vi "PicoScope6000SetupStreaming.vi"(0 "error in":errorcluster, 1 "Device Info":T2, 2 "handle in":i16, 3 "Acquisition Settings":T3={"Auto Stop"=FALSE, "Desired Sample Interval"=4, "Pre-trigger Samples"=0, "Post-trigger Samples"=1000, "Down-Sample Ratio"=1, "Down-Sample Mode"=0, "Time Units"=2} {"Time Units" items=["Nanoseconds (ns)"=2, "Microseconds (us)"=3, "Milliseconds (ms)"=4, "Seconds (s)"=5]; "Down-Sample Mode" items=["None"=0, "Aggregate"=1, "Decimate"=2, "Average"=4]}, 4 "Buffer and Transfer Settings":T1={"startIndex"=0, "Samples"=1000000, "Down Sample Ratio"=1, "Down-Sample Mode"=0} {"Down-Sample Mode" items=["None"=0, "Aggregate"=1, "Decimate"=2, "Average"=4]; "Down Sample Ratio" step=1; "Samples" format="%_6p"}, 5 "enabled array":i16[](array[numeric]), 10 "Pointers In":u64[][](array[numeric])) -> (11 "Pointer array":u64[][](array[numeric]), 14 "error out":errorcluster, 16 "handle out":i16, 17 "Sample Interval":u32, 19 "sampleIntervalTimeUnits":u32)   [LabVIEW 2016]
doc: "Set up the data buffers and calls RunStreaming to start the device streaming.\nData will be copied from the driver buffers into the corresponding application buffers using the wrapper dll."
uses:
  ps6000.dll
  ps6000Wrap.dll
panel:
  # "Overview Buffer Size is the size of the temporary buffers used to\nstore data before returning it to the application."
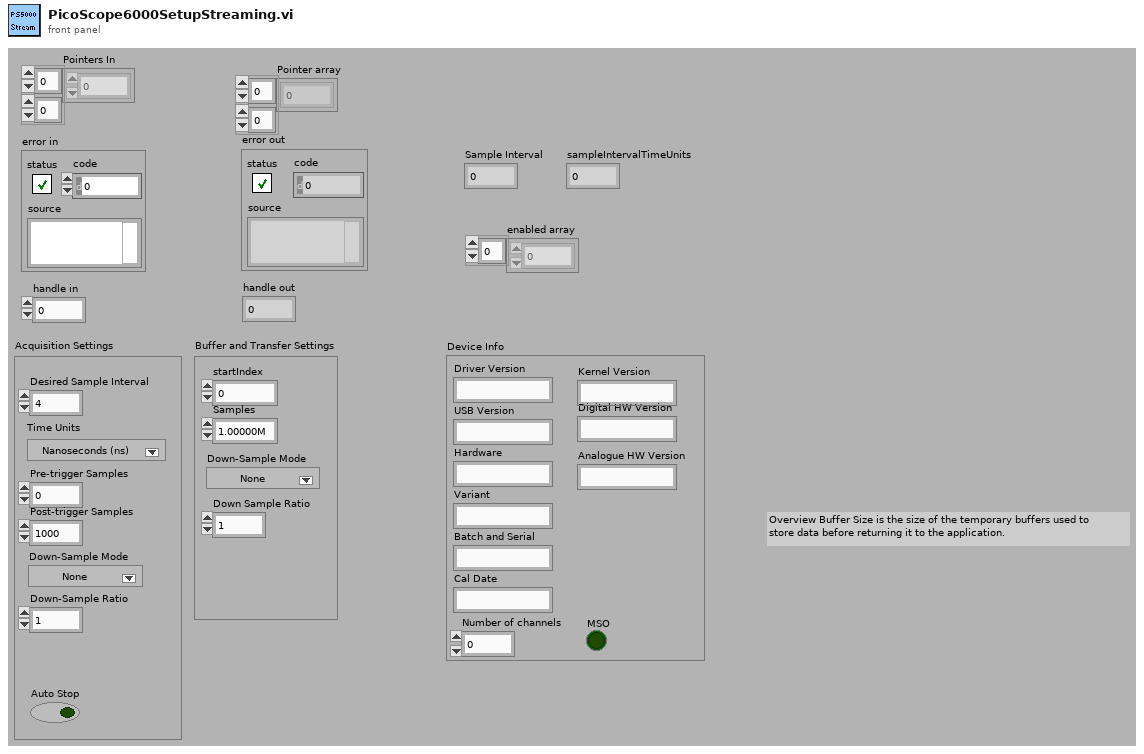
[diagram p1: front panel]
types:
  T1 = cluster{"startIndex":u64, "Samples":u64, "Down Sample Ratio":u64, "Down-Sample Mode":u32}
  T2 = cluster{"Driver Version":string, "USB Version":string, "Hardware":string, "Variant":string, "Batch and Serial":string, "Cal Date":string, "Kernel Version":string, "Digital HW Version":string, "Analogue HW Version":string, "MSO":bool, "Number of channels":i16}
  T3 = cluster{"Auto Stop":bool, "Desired Sample Interval":u32, "Pre-trigger Samples":u32, "Post-trigger Samples":u32, "Down-Sample Ratio":u32, "Down-Sample Mode":i32, "Time Units":u32}
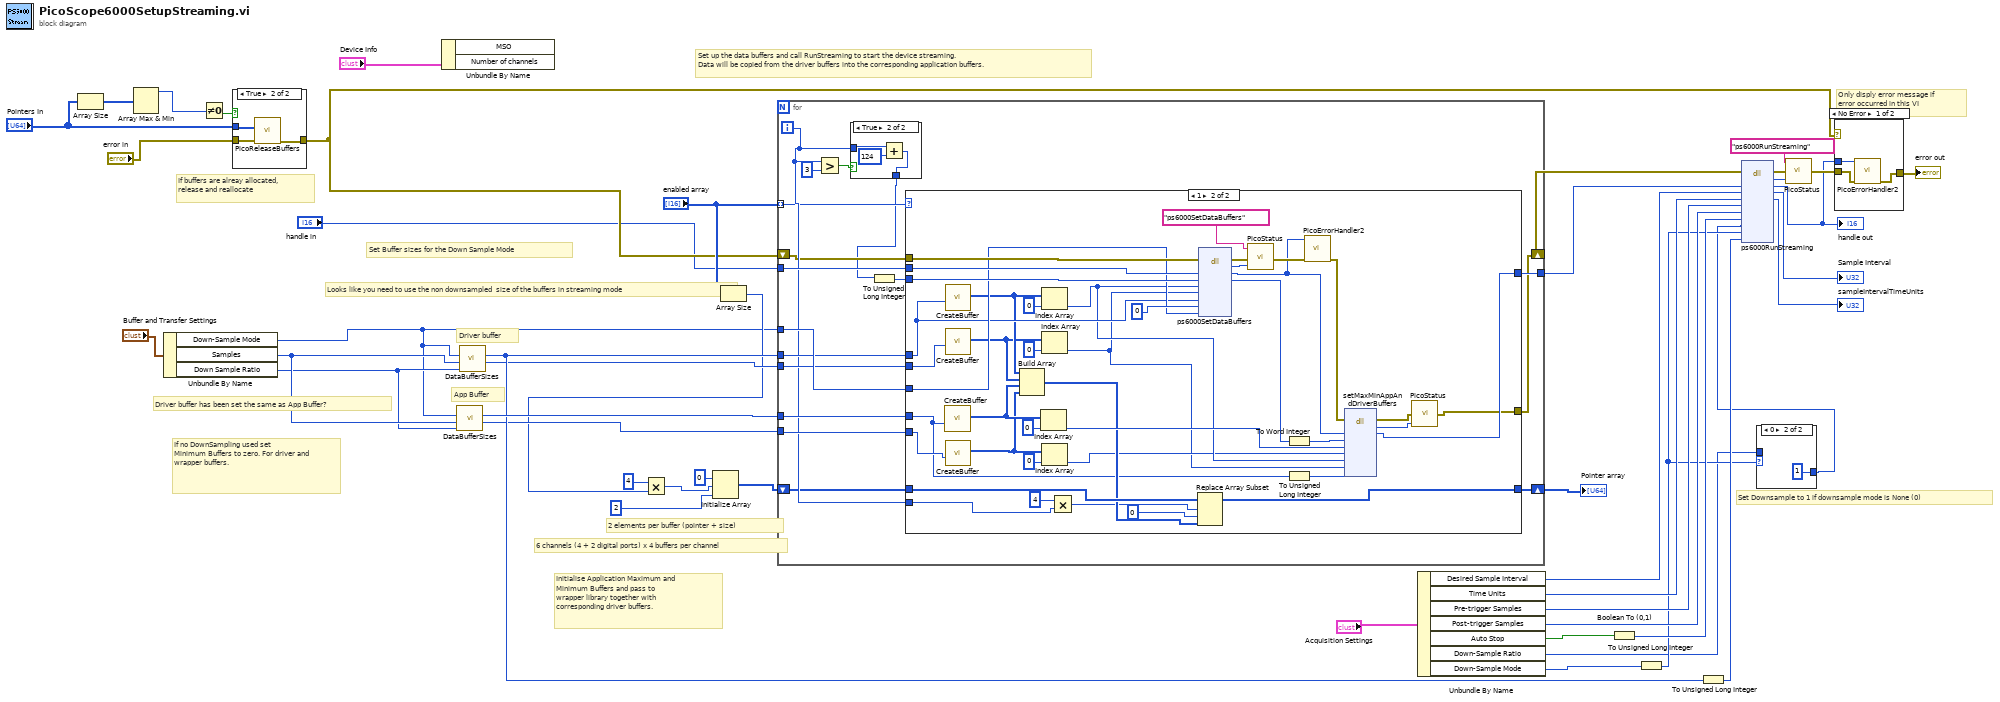
[diagram p0: block diagram]
diagram:
  # "Set Downsample to 1 if downsample mode is None (0)"
  # "Looks like you need to use the non downsampled  size of the buffers in streaming mode"
  # "If buffers are alreay allocated,\nrelease and reallocate"
  # "2 elements per buffer (pointer + size)"
  # "6 channels (4 + 2 digital ports) x 4 buffers per channel"
  # "App Buffer"
  # "Driver buffer"
  # "Driver buffer has been set the same as App Buffer?"
  # "Set Buffer sizes for the Down Sample Mode"
  # "If no DownSampling used set \nMinimum Buffers to zero. For driver and wrapper buffers."
  # "Initialise Application Maximum and\nMinimum Buffers and pass to \nwrapper library together with corresponding driver buffers."
  # "Only disply error message if\nerror occurred in this VI"
  # "Set up the data buffers and call RunStreaming to start the device streaming.\nData will be copied from the driver buffers into the corresponding application buffers."
  n1 = Array Size(array="Pointers In") -> (size(s)=w9:i32[])
  n2 = Array Max & Min(array=w9) -> (max value=w8:i32)  [unwired: 3 out]
  n3 = Unbundle By Name("Buffer and Transfer Settings") -> ("Down-Sample Mode"=w6:u32, "Samples"=w30:u64, "Down Sample Ratio"=w29:u64)
  n4 = Not Equal To 0?(x=w8) -> (x != 0?=w14:bool)
  n5 = case shown="True" w14 {
    tunnel: "Pointers In" -> [_ w48]
    tunnel: "error in" -> [w47 w49]
    tunnel: [w47 w50] -> w2
    frame False {
    }
    frame True {
      n6 = call "PicoReleaseBuffers.vi"("error in (no error)"=w49, "Pointer array"=w48) -> ("error out"=w50:errorcluster)  [unwired: 9 in]
    }
  }
  n7 = Unbundle By Name("Device Info") -> ()  [unwired: 2 out]
  n8 = call "DataBufferSizes.vi"("Down Sample Ratio"=w29, "Number of Samples"=w30, "Down-Sample Mode"=w6) -> ("min Buffer Size"=w25:i32, "Max Buffer Size"=w28:i32)  [unwired: 7 in]
  n9 = call "DataBufferSizes.vi"("Down Sample Ratio"=w29, "Number of Samples"=w30, "Down-Sample Mode"=w6) -> ("min Buffer Size"=w26:i32, "Max Buffer Size"=w27:i32)  [unwired: 7 in]
  n10 = Array Size(array="enabled array") -> (size(s)=w18:i32)
  n11 = Multiply(x=4, y=w18) -> (x*y=w19:i32)
  n12 = Initialize Array(u64 0 ("element"), w19, 2 ("dimension size")) -> (w10:u64[][])
  n13 = for {
    tunnel: "enabled array" -> [w56] mode=indexing
    tunnel: "handle in" -> [w67]
    tunnel: w6 -> [w66]
    tunnel: w28 -> [w65]
    tunnel: w27 -> [w64]
    tunnel: w26 -> [w63]
    tunnel: w25 -> [w62]
    tunnel: [w57] -> w21
    shift-right: [w55] -> w15
    shift-left: w2 -> [w54]
    shift-right: [w61] -> w24
    shift-left: w10 -> [w53]
    i -> [w58]
    n14 = Greater?(x=w58, y=3) -> (0:w59:bool)
    n15 = case shown="True" w59 {
      tunnel: [w68 w69] -> w51
      tunnel: w58 -> [w68 w71]
      frame False {
      }
      frame True {
        n16 = Add(x=w71, y=124) -> (x+y=w69:i32)
      }
    }
    n17 = To Unsigned Long Integer(number=w51) -> (unsigned 32bit integer=w52:u32)
    n18 = case shown="1" w56 {
      tunnel: w67 -> [w73 w115]
      tunnel: w54 -> [w72 w114]
      tunnel: w52 -> [_ w107]
      tunnel: w65 -> [_ w77]
      tunnel: w64 -> [_ w97]
      tunnel: w63 -> [_ w100]
      tunnel: w62 -> [_ w99]
      tunnel: w66 -> [_ w98]
      tunnel: w53 -> [w74 w91]
      tunnel: [w74 w90] -> w61
      tunnel: w58 -> [_ w87]
      tunnel: [w73 w83] -> w57
      tunnel: [w72 w82] -> w55
      frame 0, Default {
      }
      frame 1 {
        n19 = call "CreateBuffer.vi"("Buffer size"=w77) -> ("Pointer and BufferSize"=w93:u64[])  [unwired: 9 in, 1 out]
        n20 = call "CreateBuffer.vi"("Buffer size"=w97) -> ("Pointer and BufferSize"=w95:u64[])  [unwired: 9 in, 1 out]
        n21 = call "CreateBuffer.vi"("Buffer size"=w100) -> ("Pointer and BufferSize"=w94:u64[])  [unwired: 9 in, 1 out]
        n22 = call "CreateBuffer.vi"("Buffer size"=w99) -> ("Pointer and BufferSize"=w92:u64[])  [unwired: 9 in, 1 out]
        n23 = Build Array(w95, w94, w93, w92) -> (w86:u64[][])
        n24 = Index Array(array=w93, index=0) -> (element=w96:u64)
        n25 = Index Array(array=w95, index=0) -> (element=w89:u64)
        n26 = Index Array(array=w94, index=0) -> (element=w75:u64)
        n27 = Index Array(array=w92, index=0) -> (element=w76:u64)
        n28 = Multiply(x=4, y=w87) -> (x*y=w85:i32)
        n29 = Replace Array Subset(array=w91, new element=w86, index (row)=w85, index (col)=0 ("disabled index (row)")) -> (w90:u64[][])
        n30 = dll-call lib="ps6000.dll" fn="ps6000SetDataBuffers" ("ps3000.dll:_ps3000_open_unit@0")(error in=w114, "handle"=w115, "channel"=w107, "bufferMax"=w89, "bufferMin"=w75, "bufferLth"=w97, "segmentIndex"=u32 0, "downSampleRatioMode"=w98) -> (error out=w112:errorcluster, "PICO_STATUS"=w113:u32, "handle"=w79:i16, "channel"=w108:u32)  [unwired: 7 in, 1 out]
        n31 = call "PicoStatus.vi"("PICO STATUS"=w113, "error in"=w112, "source"="ps6000SetDataBuffers") -> ("error out"=w81:errorcluster)
        n32 = To Word Integer(number=w108) -> (16bit integer=w109:i16)
        n33 = To Unsigned Long Integer(number=w77) -> (unsigned 32bit integer=w78:u32)
        n34 = call "PicoErrorHandler2.vi"("error in (no error)"=w81, "handle In"=w79) -> ("error out"=w80:errorcluster)  [unwired: 9 in]
        n35 = dll-call lib="ps6000Wrap.dll" fn="setMaxMinAppAndDriverBuffers"(error in=w80, "handle"=w79, "channel"=w109, "appMaxBuffer"=w96, "appMinBuffer"=w76, "driverMaxBuffer"=w89, "driverMinBuffer"=w75, "bufferLength"=w78) -> (error out=w106:errorcluster, "status"=w105:i16, "handle"=w83:i16)  [unwired: 8 in, 1 out]
        n36 = call "PicoStatus.vi"("PICO STATUS"=w105, "error in"=w106) -> ("error out"=w82:errorcluster)  [unwired: 1 in]
      }
    }
  }
  "Pointer array" <- w24
  n37 = Unbundle By Name("Acquisition Settings") -> ("Desired Sample Interval"=w39:u32, "Time Units"=w33:u32, "Pre-trigger Samples"=w38:u32, "Post-trigger Samples"=w37:u32, "Auto Stop"=w36:bool, "Down-Sample Ratio"=w4:u32, "Down-Sample Mode"=w34:i32)
  n38 = Boolean To (0,1)(Boolean=w36) -> (0, 1=w40:i16)
  n39 = To Unsigned Long Integer(number=w34) -> (unsigned 32bit integer=w5:u32)
  n40 = To Unsigned Long Integer(number=w27) -> (unsigned 32bit integer=w7:u32)
  n41 = case shown="0" w5 {
    tunnel: [w116 u32 1 ("Down-Sample Ratio")] -> w3
    tunnel: w4 -> [w116 _]
    frame Default {
    }
    frame 0 {
    }
  }
  n42 = dll-call lib="ps6000.dll" fn="ps6000RunStreaming" ("ps5000a.dll:_ps3000_open_unit@0")(error in=w15, "handle"=w21, "sampleInterval"=w39, "sampleIntervalTimeUnits"=w33, "maxPreTriggerSamples"=w38, "maxPostTriggerSamples"=w37, "autoStop"=w40, "downSampleRatio"=w3, "downSampleRatioMode"=w5, "overviewBufferSize"=w7) -> (error out=w44:errorcluster, "PICO_STATUS"=w45:u32, "handle"=w11:i16, "sampleInterval"=→"Sample Interval":u32, "sampleIntervalTimeUnits"=→"sampleIntervalTimeUnits":u32)  [unwired: 8 in, 1 out]
  "handle out" <- w11
  n43 = call "PicoStatus.vi"("PICO STATUS"=w45, "error in"=w44, "source"="ps6000RunStreaming") -> ("error out"=w42:errorcluster)
  n44 = case shown="No Error" w2 {
    tunnel: [w119 w121] -> w46
    tunnel: w42 -> [w120 w121]
    tunnel: w11 -> [w118 _]
    frame No Error {
      n45 = call "PicoErrorHandler2.vi"("error in (no error)"=w120, "handle In"=w118) -> ("error out"=w119:errorcluster)  [unwired: 9 in]
    }
    frame Error {
    }
  }
  "error out" <- w46
